vi "Documentation.vi"   [LabVIEW 2019, in "Instrument.Element2.lvclass"]
uses:
  Instrument.Element2.lvclass
  Typedefs/Instrument.Element2.Commands--Enum.ctl
  Typedefs/Instrument.Element2.getAll--Cluster.ctl
  Typedefs/Instrument.Element2.Configuration--Cluster.ctl
  <userlib>/LevyLab/Instrument Framework/SMOs/Instrument/Instrument.lvclass
  <vilib>/JKI/JKI SMO/SMO/SMO.lvclass
  C:/Program Files (x86)/National Instruments/LabVIEW 2019/user.lib/LevyLab/Instrument Framework/Instrument Types/VSource/Instrument.VSource.lvclass
  C:/Program Files (x86)/National Instruments/LabVIEW 2019/user.lib/LevyLab/Instrument Framework/SMOs/Instrument/Instrument.lvclass
  C:/Program Files (x86)/National Instruments/LabVIEW 2019/vi.lib/JKI/JKI SMO/SMO/SMO.lvclass
  Instrument UI.Element2/Instrument UI.Element2.lvclass
  <userlib>/LevyLab/Instrument Framework/SMOs/Instrument UI/Instrument UI.lvclass
  <vilib>/JKI/JKI SMO/SMO.UI/SMO.UI.lvclass
  C:/Program Files (x86)/National Instruments/LabVIEW 2019/user.lib/LevyLab/Instrument Framework/SMOs/Instrument UI/Instrument UI.lvclass
  C:/Program Files (x86)/National Instruments/LabVIEW 2019/vi.lib/JKI/JKI SMO/SMO.UI/SMO.UI.lvclass
  Instrument UI.Element2/Instrument UI.Element2.UI--Cluster.ctl
  5668a913-f6fa-4c5c-afc1-26bd51db9186.vi
  6b6eed95-6fc9-4500-bd2e-bd5a66c15f93.vi
types:
  T1 = typedef "Instrument.Element2.lvclass/Instrument.Element2.Configuration--Cluster.ctl" = cluster{"Example Setting 1":dbl}
  T2 = typedef "Instrument.Element2.lvclass/Instrument.Element2.getAll--Cluster.ctl" = cluster{"Power":dbl}
  T3 = typedef "Instrument.Element2.lvclass/Instrument.Element2.Commands--Enum.ctl" = enum16{"command0", "command1", "command2"}
  T4 = typedef "Instrument UI.Element2.lvclass/Instrument UI.Element2.UI--Cluster.ctl" = cluster{"Parameter":dbl, "Parameter 2":string}
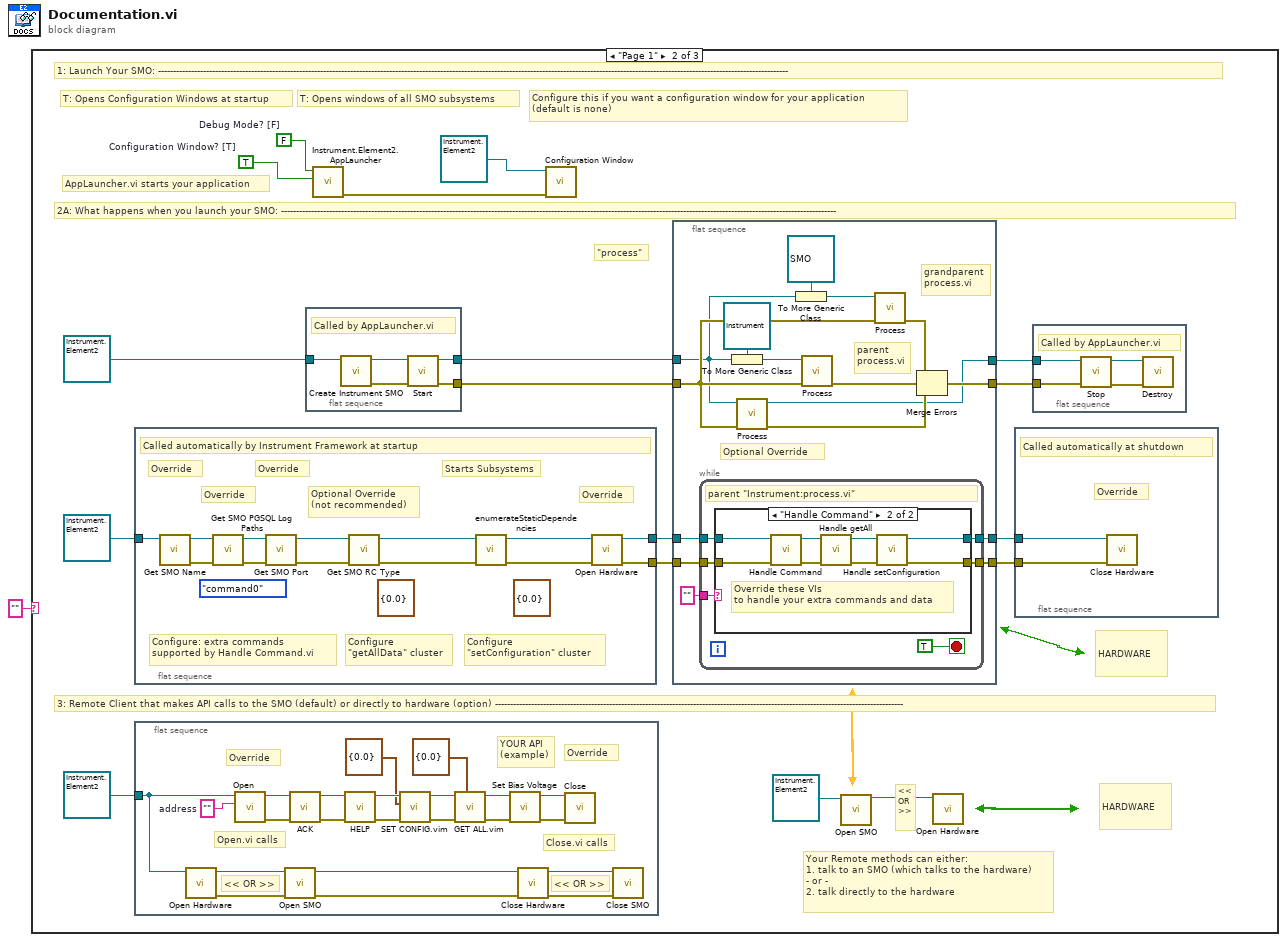
[diagram p0: block diagram]
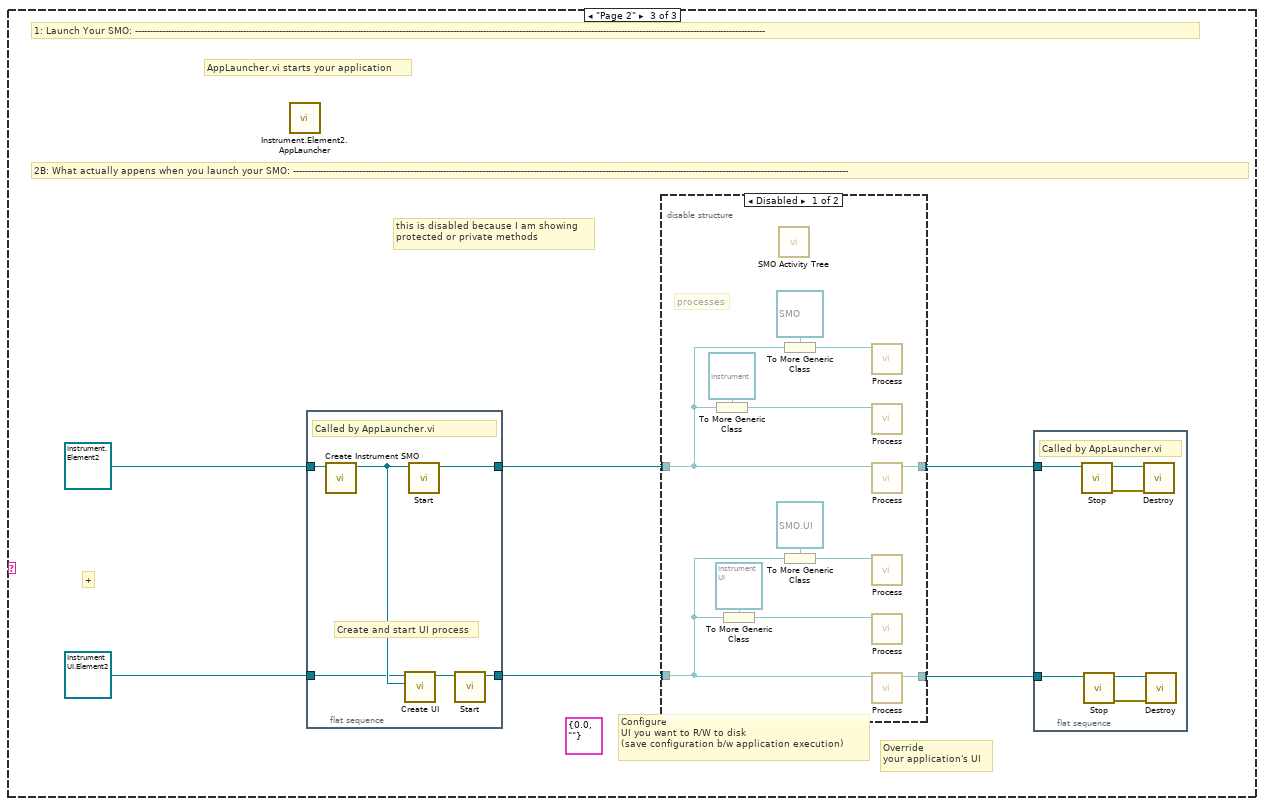
[diagram p4: hidden frame]
diagram:
  n1 = case shown="\"Page 1\"" "" {
    frame Default {
    }
    frame "Page 1" {
      w17 = TRUE  # Configuration Window? [T]
      w18 = FALSE  # Debug Mode? [F]
      # "\"process\""
      # "Your Remote methods can either:\n1. talk to an SMO (which talks to the hardware)\n- or -\n2. talk directly to the hardware"
      # "<<\nOR\n>>"
      # "HARDWARE"
      # "HARDWARE"
      # "1: Launch Your SMO: ------------------------------------------------------------------------------------------------------------------------------------------------------------------------------------------------------------------"
      # "3: Remote Client that makes API calls to the SMO (default) or directly to hardware (option) ----------------------------------------------------------------------------------------------------------------------------------------"
      # "2A: What happens when you launch your SMO: -----------------------------------------------------------------------------------------------------------------------------------------------------------------------------------------"
      # "Configure this if you want a configuration window for your application\n(default is none)"
      # "AppLauncher.vi starts your application"
      # "T: Opens windows of all SMO subsystems"
      # "T: Opens Configuration Windows at startup"
      n2 = flat-sequence {
        tunnel: [w59] -> w16
        tunnel: [w58] -> w14
        tunnel: refnum<class "Instrument.Element2.lvclass"> refnum ("Instrument.Template.lvclass") -> [w57]
        frame #0 {
          (unwired) T1 {"Example Setting 1"=0.0} ("Configuration")
          (unwired) T2 {"Power"=0.0} ("getAll")
          (unwired) Instrument.Element2.Commands--Enum."command0" ("Commands")
          # "Configure\n\"setConfiguration\" cluster"
          # "Configure\n\"getAllData\" cluster"
          # "Configure: extra commands\nsupported by Handle Command.vi"
          # "Override"
          # "Starts Subsystems"
          # "Override"
          # "Override"
          # "Override"
          # "Optional Override\n(not recommended)"
          # "Called automatically by Instrument Framework at startup"
          n3 = call-dynamic "Get SMO Name.vi"("Example Instrument in"=w57) -> ("error out"=w55:errorcluster, "Example Instrument out"=w56:refnum<class "Instrument.Element2.lvclass">)  [unwired: 8 in, 1 out]
          n4 = call-dynamic "Get SMO PGSQL Log Paths.vi"("error in (no error)"=w55, "Example in"=w56) -> ("error out"=w53:errorcluster, "Example out"=w54:refnum<class "Instrument.Element2.lvclass">)  [unwired: 7 in, 1 out]
          n5 = call-dynamic "Get SMO Port.vi"("error in (no error)"=w53, "ExampleInstrument in"=w54) -> ("error out"=w60:errorcluster, "ExampleInstrument out"=w61:refnum<class "Instrument.Element2.lvclass">)  [unwired: 7 in, 1 out]
          n6 = call-dynamic "Get SMO RC Type.vi"("error in (no error)"=w60, "ExampleInstrument in"=w61) -> ("error out"=w62:errorcluster, "ExampleInstrument out"=w63:refnum<class "Instrument.Element2.lvclass">)  [unwired: 7 in, 1 out]
          n7 = call-dynamic "enumerateStaticDependencies.vi"("error in (no error)"=w62, "Instrument"=w63) -> ("error out"=w64:errorcluster, "Instrument out"=w65:refnum<class "Instrument.Element2.lvclass">)  [unwired: 7 in, 1 out]
          n8 = call-dynamic "Open Hardware.vi"("error in (no error)"=w64, "Instrument.Template in"=w65) -> ("error out"=w58:errorcluster, "Instrument.Template out"=w59:refnum<class "Instrument.Element2.lvclass">)  [unwired: 8 in]
        }
      }
      n9 = flat-sequence {
        tunnel: refnum<class "Instrument.Element2.lvclass"> refnum ("Instrument.Template.lvclass") -> [w71]
        frame #0 {
          w73 = ""  # address
          # "Close.vi calls"
          # "Open.vi calls"
          # "<< OR >>"
          # "<< OR >>"
          # "YOUR API\n(example)"
          # "Override"
          # "Override"
          n10 = call-dynamic "Open Hardware.vi"("Instrument.Template in"=w71) -> ("error out"=w66:errorcluster, "Instrument.Template out"=w70:refnum<class "Instrument.Element2.lvclass">)  [unwired: 9 in]
          n11 = call-dynamic "Open.vi"("address"=w73, "Instrument.Template in"=w71) -> ("error out"=w87:errorcluster, "Instrument.Template out"=w86:refnum<class "Instrument.Element2.lvclass">)  [unwired: 8 in]
          n12 = call <userlib>:"Open SMO.vi"("error in (no error)"=w66, "Instrument in"=w70) -> ("error out"=w67:errorcluster, "Instrument out"=w69:refnum<class "Instrument.Element2.lvclass">)  [unwired: 8 in]
          n13 = call <userlib>:"ACK.vi"("error in (no error)"=w87, "Instrument in"=w86) -> ("error out"=w85:errorcluster, "Instrument out"=w84:refnum<class "Instrument.Element2.lvclass">)  [unwired: 7 in, 1 out]
          n14 = call <userlib>:"HELP.vi"("error in (no error)"=w85, "Instrument in"=w84) -> ("error out"=w79:errorcluster, "Instrument in"=w80:refnum<class "Instrument.Element2.lvclass">)  [unwired: 7 in, 1 out]
          n15 = call "SET CONFIG.vim"("error in (no error)"=w79, "Configuration"=T1 {"Example Setting 1"=0.0}, "Instrument in"=w80) -> ("error out"=w74:errorcluster, "Instrument out"=w77:refnum<class "Instrument.Element2.lvclass">)  [unwired: 7 in]
          n16 = call "GET ALL.vim"("type"=T2 {"Power"=0.0} ("getAll"), "error in (no error)"=w74, "Instrument in"=w77) -> ("error out"=w75:errorcluster, "Instrument out"=w76:refnum<class "Instrument.Element2.lvclass">)  [unwired: 6 in, 1 out]
          n17 = call-dynamic "Set Bias Voltage.vi"("error in (no error)"=w75, "Example in"=w76) -> ("error out"=w82:errorcluster, "Example out"=w83:refnum<class "Instrument.Element2.lvclass">)  [unwired: 8 in]
          n18 = call-dynamic "Close Hardware.vi"("error in (no error)"=w67, "Instrument.Template in"=w69) -> ("error out"=w72:errorcluster, "Instrument.Template out"=w68:refnum<class "Instrument.Element2.lvclass">)  [unwired: 8 in]
          n19 = call-dynamic "Close.vi"("error in (no error)"=w82, "Instrument.Template in"=w83) -> ()  [unwired: 8 in, 2 out]
          n20 = call <userlib>:"Close SMO.vi"("error in (no error)"=w72, "Instrument in"=w68) -> ()  [unwired: 8 in, 2 out]
        }
      }
      n21 = flat-sequence {
        tunnel: [w94] -> w4
        tunnel: [w93] -> w6
        tunnel: refnum<class "Instrument.Element2.lvclass"> refnum ("Instrument.Template.lvclass") -> [w92]
        frame #0 {
          # "Called by AppLauncher.vi"
          n22 = call-dynamic "Create Instrument SMO.vi"("Instrument in"=w92) -> ("error out"=w95:errorcluster, "Instrument out"=w96:refnum<class "Instrument.Element2.lvclass">)  [unwired: 9 in]
          n23 = call <vilib>:"Start.vi"("error in (no error)"=w95, "SMO"=w96) -> ("error out"=w93:errorcluster, "SMO out"=w94:refnum<class "Instrument.Element2.lvclass">)  [unwired: 8 in]
        }
      }
      n24 = call "Instrument.Element2.AppLauncher.vi"("Configuration Window? [T]"=w17, "Debug Mode? [F]"=w18) -> ("error out"=w11:errorcluster)  [unwired: 9 in]
      n25 = call-dynamic "Configuration Window.vi"("error in (no error)"=w11, "Example Instrument in"=refnum<class "Instrument.Element2.lvclass"> refnum ("Instrument.Template.lvclass")) -> ()  [unwired: 8 in, 2 out]
      n26 = flat-sequence {
        tunnel: w16 -> [w34]
        tunnel: [w33] -> w15
        tunnel: w14 -> [w32]
        tunnel: [w31] -> w13
        tunnel: [w29] -> w7
        tunnel: w6 -> [w27]
        tunnel: [w20] -> w5
        tunnel: w4 -> [w19]
        frame #0 {
          # "Optional Override"
          # "grandparent\nprocess.vi"
          # "parent\nprocess.vi"
          n27 = while {
            tunnel: "" -> [w40]
            tunnel: w34 -> [w38]
            tunnel: [w37] -> w33
            tunnel: w32 -> [w36]
            tunnel: [w35] -> w31
            stop <- TRUE stop-if-true
            # "parent \"Instrument:process.vi\""
            n28 = case shown="\"Handle Command\"" w40 {
              tunnel: w38 -> [w42 w50]
              tunnel: [w42 w46] -> w37
              tunnel: w36 -> [w41 w49]
              tunnel: [w41 w45] -> w35
              frame Default {
              }
              frame "Handle Command" {
                # "Override these VIs\nto handle your extra commands and data"
                n29 = call-dynamic "Handle Command.vi"("error in (no error)"=w49, "Example Instrument in"=w50) -> ("error out"=w43:errorcluster, "Example Instrument out"=w48:refnum<class "Instrument.Element2.lvclass">)  [unwired: 6 in, 2 out]
                n30 = call-dynamic "Handle getAll.vi"("error in (no error)"=w43, "Example Instrument in"=w48) -> ("error out"=w44:errorcluster, "Example Instrument out"=w47:refnum<class "Instrument.Element2.lvclass">)  [unwired: 7 in, 1 out]
                n31 = call-dynamic "Handle setConfiguration.vi"("error in (no error)"=w44, "Instrument.Template in"=w47) -> ("error out"=w45:errorcluster, "Instrument.Template out"=w46:refnum<class "Instrument.Element2.lvclass">)  [unwired: 8 in]
              }
            }
          }
          n32 = To More Generic Class(target class=refnum<class "Instrument.lvclass"> refnum ("Instrument"), reference=w19) -> (generic class reference=w26:refnum<class "Instrument.lvclass">)
          n33 = call-dynamic "Process.vi"("error in"=w27, "Example Instrument"=w19) -> ("error out"=w22:errorcluster, "Example Instrument out"=w20:refnum<class "Instrument.Element2.lvclass">)  [unwired: 8 in]
          n34 = To More Generic Class(target class=refnum<class "SMO.lvclass"> refnum ("SMO"), reference=w19) -> (generic class reference=w28:refnum<class "SMO.lvclass">)
          n35 = call-dynamic "Process.vi"("error in"=w27, "Instrument"=w26) -> ("error out"=w23:errorcluster)  [unwired: 8 in, 1 out]
          n36 = call-dynamic "Process.vi"("error in"=w27, "SMO"=w28) -> ("error out"=w21:errorcluster)  [unwired: 8 in, 1 out]
          n37 = Merge Errors(w21, w23, w22) -> (w29:errorcluster)
        }
      }
      n38 = call <userlib>:"Open SMO.vi"("Instrument in"=refnum<class "Instrument.Element2.lvclass"> refnum ("Instrument.Template.lvclass")) -> ("Instrument out"=w3:refnum<class "Instrument.Element2.lvclass">)  [unwired: 9 in, 1 out]
      n39 = call-dynamic "Open Hardware.vi"("Instrument.Template in"=w3) -> ()  [unwired: 9 in, 2 out]
      n40 = flat-sequence {
        tunnel: w15 -> [w52]
        tunnel: w13 -> [w51]
        frame #0 {
          # "Override"
          # "Called automatically at shutdown"
          n41 = call-dynamic "Close Hardware.vi"("error in (no error)"=w51, "Instrument.Template in"=w52) -> ()  [unwired: 8 in, 2 out]
        }
      }
      n42 = flat-sequence {
        tunnel: w5 -> [w89]
        tunnel: w7 -> [w88]
        frame #0 {
          # "Called by AppLauncher.vi"
          n43 = call <vilib>:"Stop.vi"("error in (no error)"=w88, "SMO"=w89) -> ("error out"=w91:errorcluster, "SMO out"=w90:refnum<class "Instrument.Element2.lvclass">)  [unwired: 8 in]
          n44 = call <vilib>:"Destroy.vi"("error in (no error)"=w91, "SMO"=w90) -> ()  [unwired: 9 in, 1 out]
        }
      }
    }
    frame "Page 2" {
      (unwired) T4 {"Parameter"=0.0, "Parameter 2"=""} ("UI")
      # "this is disabled because I am showing\nprotected or private methods"
      # "Configure\nUI you want to R/W to disk\n(save configuration b/w application execution)"
      # "Override\nyour application's UI"
      # "+"
      # "1: Launch Your SMO: ------------------------------------------------------------------------------------------------------------------------------------------------------------------------------------------------------------------"
      # "2B: What actually appens when you launch your SMO: -----------------------------------------------------------------------------------------------------------------------------------------------------------------------------------------"
      # "AppLauncher.vi starts your application"
      n45 = call "Instrument.Element2.AppLauncher.vi"() -> ()  [unwired: 11 in, 1 out]
      n46 = flat-sequence {
        tunnel: [w114] -> w100
        tunnel: refnum<class "Instrument.Element2.lvclass"> refnum ("Instrument.Template.lvclass") -> [w113]
        tunnel: refnum<class "Instrument UI.Element2.lvclass"> refnum ("Instrument UI.Template.lvclass") -> [w111]
        tunnel: [w109] -> w98
        frame #0 {
          # "Create and start UI process"
          # "Called by AppLauncher.vi"
          n47 = call-dynamic "Create Instrument SMO.vi"("Instrument in"=w113) -> ("Instrument out"=w112:refnum<class "Instrument.Element2.lvclass">)  [unwired: 9 in, 1 out]
          n48 = call <userlib>:"Create UI.vi"("Instrument in"=w112, "Instrument UI"=w111) -> ("Instrument UI out"=w110:refnum<class "Instrument UI.Element2.lvclass">)  [unwired: 8 in, 1 out]
          n49 = call <vilib>:"Start.vi"("SMO"=w112) -> ("SMO out"=w114:refnum<class "Instrument.Element2.lvclass">)  [unwired: 9 in, 1 out]
          n50 = call <vilib>:"Start.vi"("SMO"=w110) -> ("SMO out"=w109:refnum<class "Instrument UI.Element2.lvclass">)  [unwired: 9 in, 1 out]
        }
      }
      n51 = disable-structure shown="Disabled" {
        disable-tunnel: [w126 w128] -> w101
        disable-tunnel: w100 -> [w125 w128]
        disable-tunnel: w98 -> [w124 w127]
        disable-tunnel: [w123 w127] -> w97
        frame Disabled {
          # "processes"
          n52 = To More Generic Class(target class=refnum<class "Instrument.lvclass"> refnum ("Instrument"), reference=w125) -> (generic class reference=w121:refnum<class "Instrument.lvclass">)
          n53 = To More Generic Class(target class=refnum<class "Instrument UI.lvclass"> refnum ("Instrument UI"), reference=w124) -> (generic class reference=w117:refnum<class "Instrument UI.lvclass">)
          n54 = call <vilib>:"SMO Activity Tree.vi"() -> ()  [unwired: 12 in]
          n55 = To More Generic Class(target class=refnum<class "SMO.lvclass"> refnum ("SMO"), reference=w125) -> (generic class reference=w122:refnum<class "SMO.lvclass">)
          n56 = To More Generic Class(target class=refnum<class "SMO.UI.lvclass"> refnum ("SMO.UI"), reference=w124) -> (generic class reference=w115:refnum<class "SMO.UI.lvclass">)
          n57 = call-dynamic "Process.vi"("SMO"=w122) -> ()  [unwired: 9 in, 2 out]
          n58 = call-dynamic "Process.vi"("Instrument"=w121) -> ()  [unwired: 9 in, 2 out]
          n59 = call-dynamic "Process.vi"("Example Instrument"=w125) -> ("Example Instrument out"=w126:refnum<class "Instrument.Element2.lvclass">)  [unwired: 9 in, 1 out]
          n60 = call-dynamic "Process.vi"("SMO.UI"=w115) -> ()  [unwired: 9 in, 2 out]
          n61 = call-dynamic "Process.vi"("Instrument UI in"=w117) -> ()  [unwired: 9 in, 2 out]
          n62 = call-dynamic "Process.vi"("Example Instrument UI"=w124) -> ("Example Instrument UI out"=w123:refnum<class "Instrument UI.Element2.lvclass">)  [unwired: 9 in, 1 out]
        }
        frame Enabled {
        }
      }
      n63 = flat-sequence {
        tunnel: w101 -> [w106]
        tunnel: w97 -> [w104]
        frame #0 {
          # "Called by AppLauncher.vi"
          n64 = call <vilib>:"Stop.vi"("SMO"=w106) -> ("error out"=w108:errorcluster, "SMO out"=w107:refnum<class "Instrument.Element2.lvclass">)  [unwired: 9 in]
          n65 = call <vilib>:"Stop.vi"("SMO"=w104) -> ("error out"=w105:errorcluster, "SMO out"=w103:refnum<class "Instrument UI.Element2.lvclass">)  [unwired: 9 in]
          n66 = call <vilib>:"Destroy.vi"("error in (no error)"=w108, "SMO"=w107) -> ()  [unwired: 9 in, 1 out]
          n67 = call <vilib>:"Destroy.vi"("error in (no error)"=w105, "SMO"=w103) -> ()  [unwired: 9 in, 1 out]
        }
      }
    }
  }
